vi "Add Filters.vi"(8 "error in (no error)":errorcluster, 10 "Filters":refnum<class "Filter.lvclass">[](array[class]), 11 "Bus Monitor in":refnum<class "Bus Monitor.lvclass">) -> (0 "error out":errorcluster, 3 "Bus Monitor out":refnum<class "Bus Monitor.lvclass">)   [LabVIEW 2020, in "BCI-1553 API.lvlib" / "Bus Monitor.lvclass"]
doc: "Adds Filters to this Bus Monitor. Each Filter should have a unique ID. If two Filters have colliding IDs, the newest Filter will take priority and will replace the existing one."
uses:
  Bus Monitor.lvclass
  Filters/Filter/Filter.lvclass
  Bus Monitor.lvclass/Bus Monitor.ctl
  Dependencies/Registry/Registry.lvclass/Registry.ctl
  Dependencies/Registry/Add Entry.vi
  Dependencies/Registry/Registry.lvclass
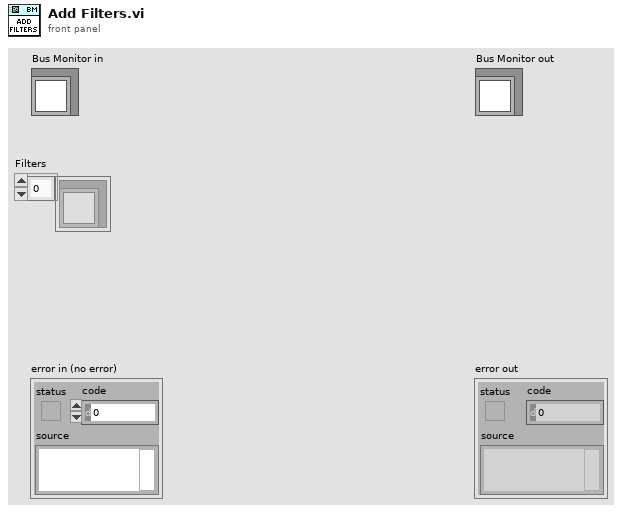
[diagram p1: front panel]
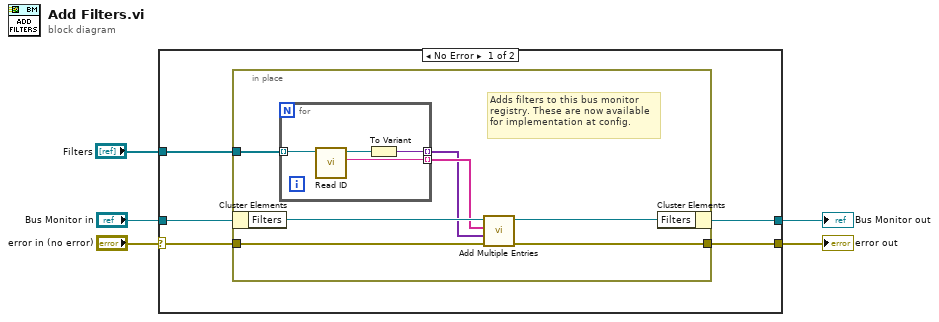
[diagram p0: block diagram]
diagram:
  n1 = case shown="No Error" "error in (no error)" {
    selector: "error in (no error)" -> [w7 w23]
    tunnel: [w8 w23] -> w3
    tunnel: [w9 w22] -> w2
    tunnel: "Bus Monitor in" -> [w10 w22]
    tunnel: "Filters" -> [w6 _]
    frame No Error {
      n2 = in-place {
        in-place-border: [w15] -> w8
        in-place-border: w7 -> [w14]
        in-place-border: w6 -> [w13]
        # "Adds filters to this bus monitor\nregistry. These are now available\nfor implementation at config."
        n3 = in-place-cluster #1(w10) -> ("Filters"=w17:refnum<class "Registry.lvclass">)
        n4 = for {
          tunnel: w13 -> [w20] mode=indexing
          tunnel: [w19] -> w12 mode=indexing
          tunnel: [w21] -> w11 mode=indexing
          n5 = call-dynamic "Read ID.vi"("Filter in"=w20) -> ("ID"=w19:string, "Filter out"=w18:refnum<class "Filter.lvclass">)  [unwired: 8 in, 1 out]
          n6 = To Variant(anything=w18) -> (Variant=w21:variant)
        }
        n7 = call "Add Multiple Entries.vi"("error in (no error)"=w14, "Values"=w11, "Keys"=w12, "Registry in"=w17) -> ("error out"=w15:errorcluster, "Registry out"=w16:refnum<class "Registry.lvclass">)  [unwired: 5 in, 1 out]
        n8 = in-place-cluster #1("Filters"=w16) -> (w9:refnum<class "Bus Monitor.lvclass">)
      }
    }
    frame Error {
    }
  }
  "error out" <- w3
  "Bus Monitor out" <- w2
